vi "oax_Compute Order Resolution.vi"(9 "actual max order":dbl, 10 "order resolution":dbl=0.1 min=0.0 format="%.3f", 11 "block size":i32=1024 min=2) -> (2 "actual order resolution\n[order]":dbl=2.0, 3 "block size out":i32=1024 min=2)   [LabVIEW 2017]
doc: "Determines the block size used to compute the order-power spectrum of the even-angle-spaced signal."
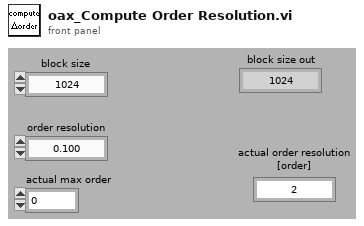
[diagram p1: front panel]
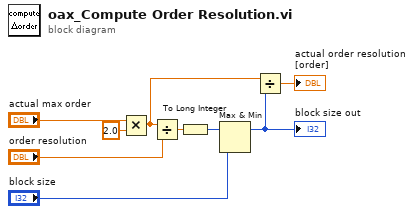
[diagram p0: block diagram]
diagram:
  n1 = Multiply(x="actual max order", y=2.0) -> (x*y=w4:dbl)
  n2 = Divide(x=w4, y="order resolution") -> (x/y=w6:dbl)
  n3 = To Long Integer(number=w6) -> (32bit integer=w1:i32)
  n4 = Max & Min(x=w1, y="block size") -> (max(x,y)=w3:i32)  [unwired: 1 out]
  "block size out" <- w3
  n5 = Divide(x=w4, y=w3) -> (x/y=→"actual order resolution\n[order]":dbl)
